vi "DMMsTest.vi"() -> ()   [LabVIEW 2017]
uses:
  DMMsData.lvclass
panel:
  out "LastData":dbl[](array[numeric])
  out "DeviceActive?":bool[](array[boolean])
  out "XY Graph":T1(graph)
  in  "DMMsConfig":T2(array[cluster])
  out "DMMsLabels":string[](array[string])
  in  "stop":bool
  out "error out":errorcluster
  out "cycle #":i32
  out "RUN indicator":string
  in  "RUN label":string
  in  "base path":path
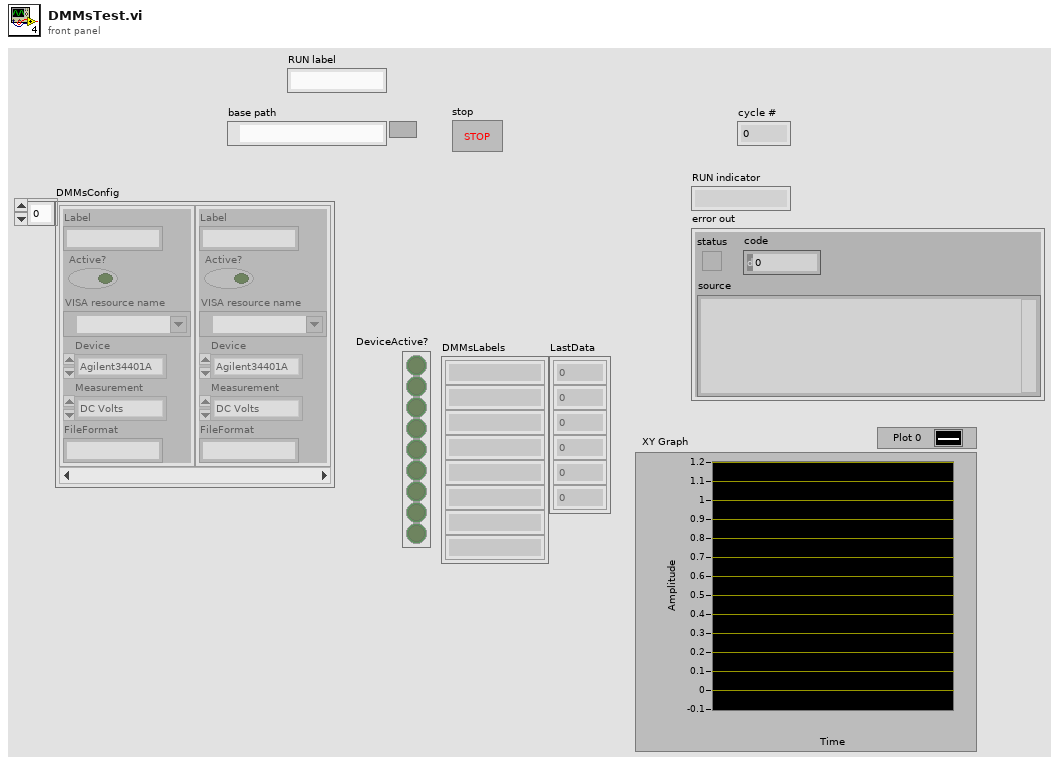
[diagram p1: front panel]
types:
  T1 = cluster{"TimeArray":timestamp[], "DataArray":dbl[]}[]
  T2 = cluster{"Label":string, "Active?":bool, "VISA resource name":refnum<visa-resource-name>, "Device":enum16{"Agilent34401A", "ADCMT7351", "HP3478A"}, "Measurement":enum16{"DC Volts", "DC Currents", "2-Wire Resistance", "4-Wire Resistance"}, "FileFormat":string}[]
  T3 = cluster{"TimeArray":timestamp[], "DataArray":dbl[]}
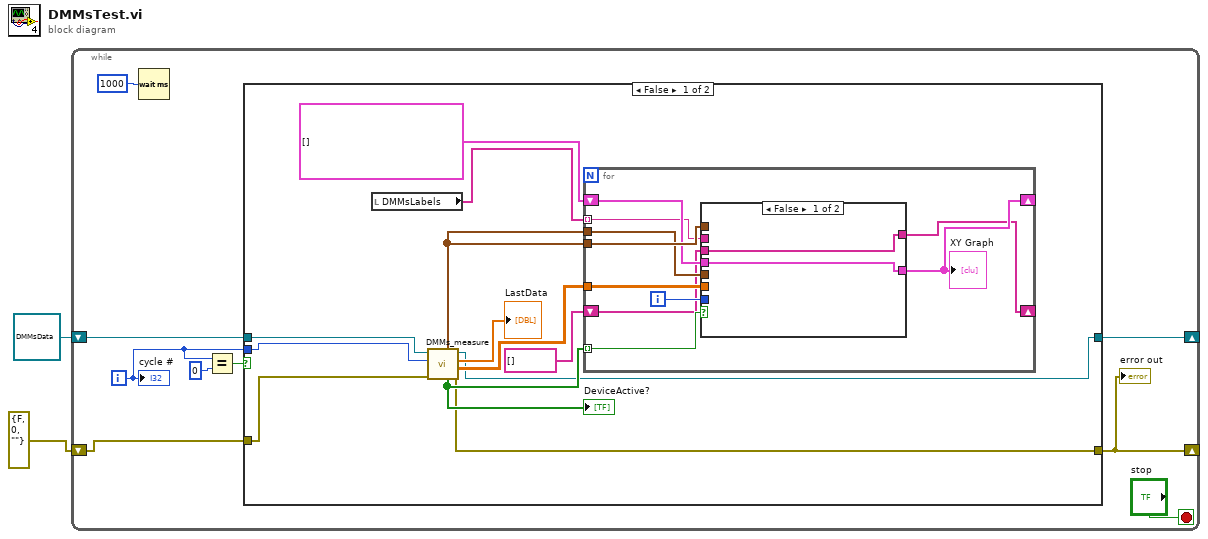
[diagram p0: block diagram]
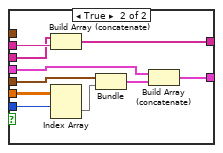
[diagram p2: hidden frame]
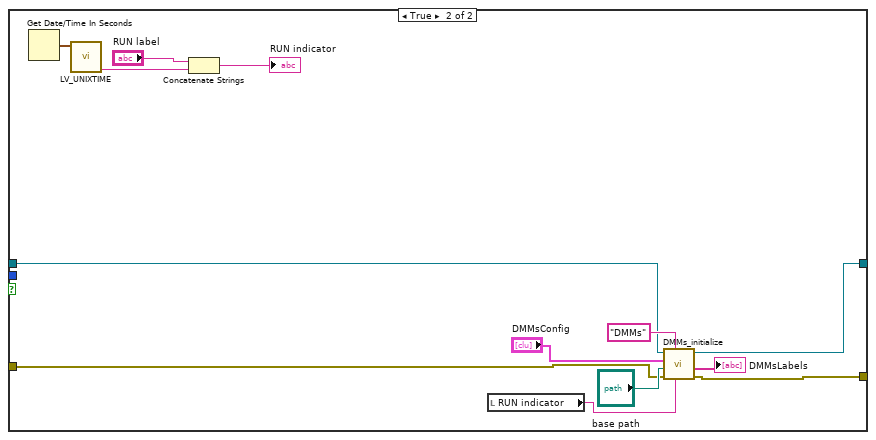
[diagram p3: hidden frame]
diagram:
  n1 = while {
    shift-right: [w3] -> _
    shift-left: refnum<class "DMMsData.lvclass"> refnum ("DMMsData in") -> [w7]
    shift-right: [w5] -> _
    shift-left: errorcluster {"status"=FALSE, "code"=0, "source"=""} ("error in (no error)") -> [w4]
    i -> [w8]
    stop <- "stop" stop-if-true
    n2 = Wait (ms)(milliseconds to wait=u32 1000) -> ()  [unwired: 1 out]
    n3 = Equal?(x=w8, y=0) -> (x = y?=w6:bool)
    n4 = case shown="False" w6 {
      tunnel: w8 -> [w16 _]
      tunnel: w7 -> [w15 w48]
      tunnel: [w14 w49] -> w5
      tunnel: w4 -> [w12 w47]
      tunnel: [w13 w46] -> w3
      frame False {
        n5 = local read "DMMsLabels"() -> (w19:string[])
        n6 = call-dynamic "DMMs_measure.vi"("error in (no error)"=w12, "MeasurementIndex"=w16, "DMMsData in"=w15) -> ("error out"=w14:errorcluster, "DataArray"=w23:dbl[][], "LastData"=→"LastData":dbl[], "DMMsData out"=w13:refnum<class "DMMsData.lvclass">, "DeviceActive?"=w20:bool[], "TimeArray"=w22:timestamp[])  [unwired: 3 in]
        "DeviceActive?" <- w20
        n7 = for {
          tunnel: w22 -> [w33]
          shift-right: [w28] -> _
          shift-left: T1 [] -> [w32]
          tunnel: w23 -> [w31]
          tunnel: w22 -> [w30]
          tunnel: w20 -> [w27] mode=indexing
          shift-right: [w26] -> _
          shift-left: string[] [] -> [w24]
          tunnel: w19 -> [w25] mode=indexing
          i -> [w29]
          n8 = case shown="False" w27 {
            tunnel: w33 -> [_ _]
            tunnel: [w35 w45] -> w28
            tunnel: w32 -> [w35 w39]
            tunnel: w31 -> [_ w44]
            tunnel: w30 -> [_ w43]
            tunnel: w29 -> [_ w41]
            tunnel: [w34 w38] -> w26
            tunnel: w25 -> [_ w37]
            tunnel: w24 -> [w34 w36]
            frame False {
            }
            frame True {
              n9 = Build Array (concatenate)(w36, w37) -> (w38:string[])
              n10 = Index Array(array=w44, index (row)=w41) -> (element=w42:dbl[])  [unwired: 1 in]
              n11 = Bundle("TimeArray"=w43, "DataArray"=w42) -> (w40:T3)  [unwired: 1 in]
              n12 = Build Array (concatenate)(w39, w40) -> (w45:T1)
            }
          }
          "XY Graph" <- w28
        }
      }
      frame True {
        n13 = Get Date/Time In Seconds() -> (seconds since 1Jan1904=w55:timestamp)
        n14 = call "LV_UNIXTIME.vi"("current time"=w55) -> ("date/time string"=w56:string)  [unwired: 9 in, 1 out]
        n15 = Concatenate Strings("RUN label", w56) -> (→"RUN indicator":string)
        n16 = local read "RUN indicator"() -> (w51:string)
        n17 = call-dynamic "DMMs_initialize.vi"("RunIdentifier"=w51, "InstName"="DMMs", "error in (no error)"=w47, "base path"="base path", "DMMsConfig"="DMMsConfig", "DMMsData in"=w48) -> ("error out"=w49:errorcluster, "DMMsLabels"=→"DMMsLabels":string[], "DMMsData out"=w46:refnum<class "DMMsData.lvclass">)  [unwired: 3 in]
      }
    }
    "error out" <- w5
    "cycle #" <- w8
  }
